vi "tempsave.vi"() -> ()   [LabVIEW 2014]
uses:
  <vilib>/rvi/DataTransferAndStorage/Container/XNode/niFpgaContainer.xnode
  <vilib>/rvi/FIFO/Fifo_Resource/niFpgaFifoEmulationRefIn.vi
  FPGA Function.ctl
panel:
  in  "PosVal 2":u32
  in  "SerialFunction 2":T1
  out "NOBWrite 2":i32
  in  "Delay W/R 2":u32=4
  out "Pos 2":u32
  out "Position":i32
  out "Pos 1":u32
  in  "PosVal":u32
  in  "SerialFunction":T1
  out "PresentPos":u64[](array[numeric])
  out "NOBWrite":i32
  in  "Delay W/R":u32=550
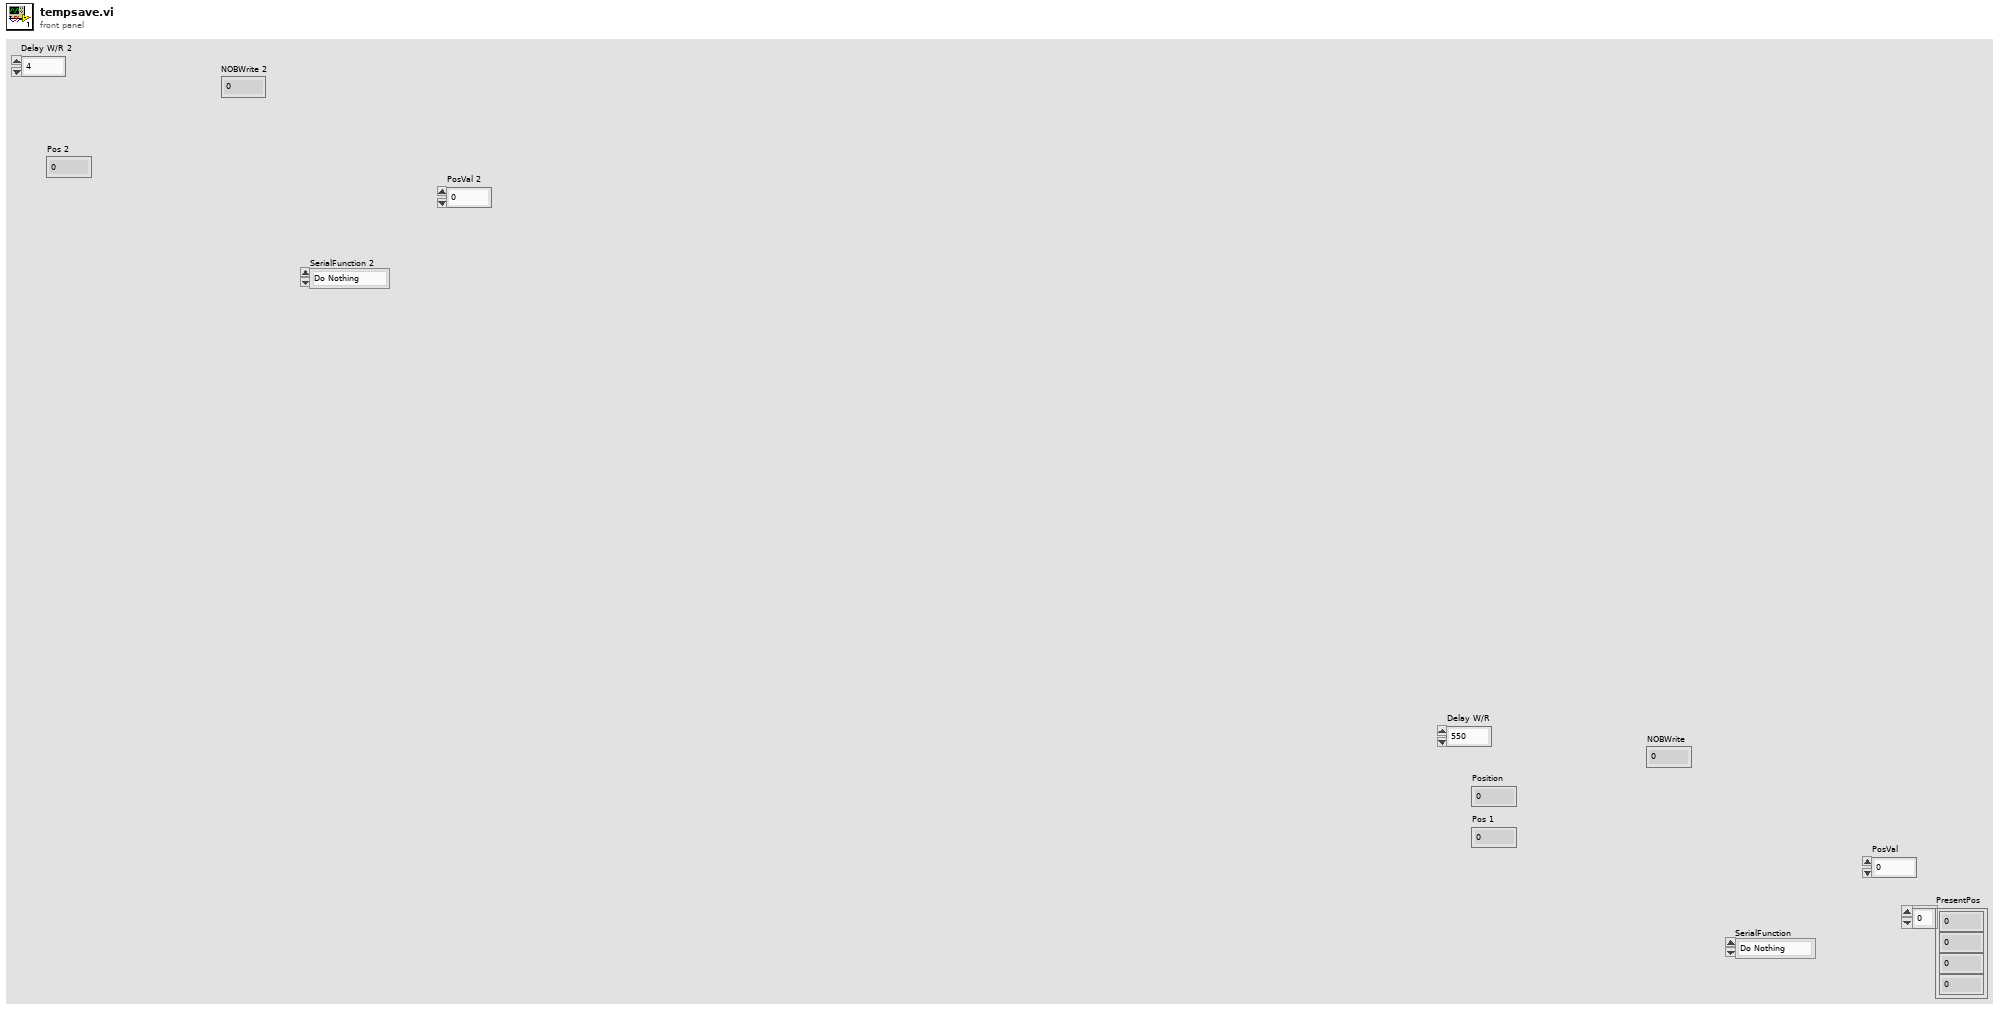
[diagram p1: front panel]
types:
  T1 = typedef "FPGA Function.ctl" = enum16{"Do Nothing", "Write", "Read"}
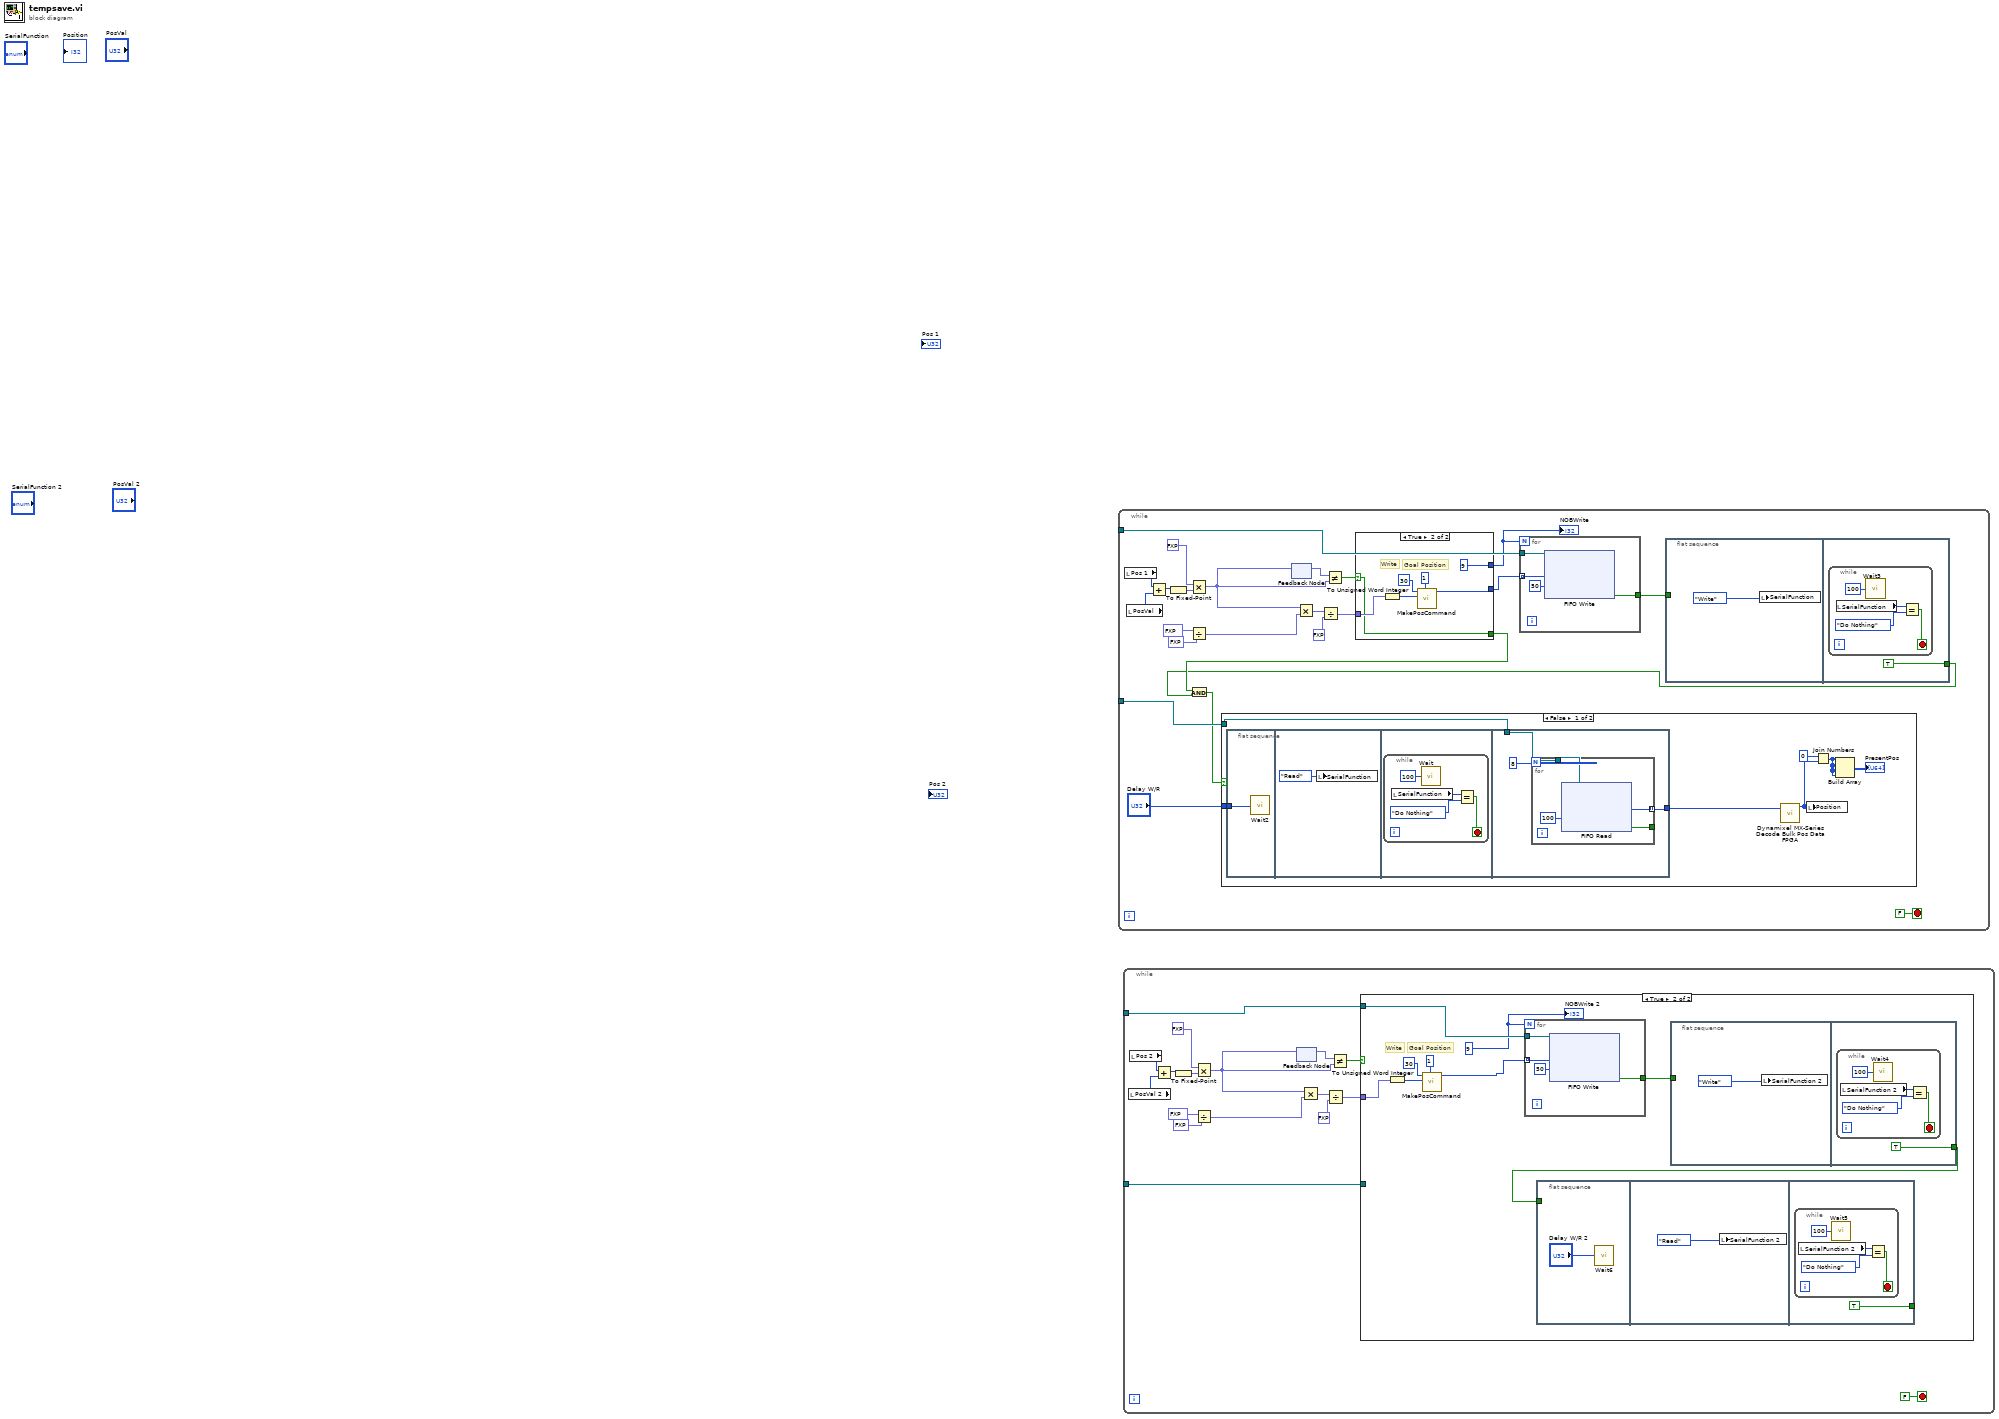
[diagram p0: block diagram]
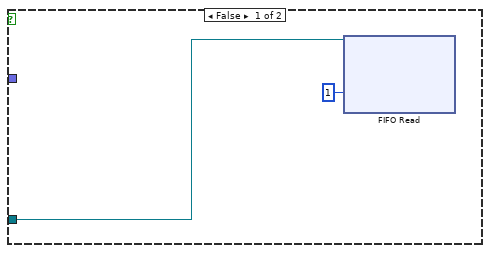
[diagram p2: hidden frame]
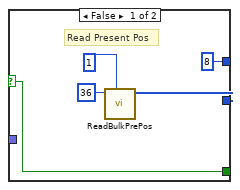
[diagram p4: hidden frame]
diagram:
  n1 = while {
    tunnel: _ -> [w9]
    tunnel: _ -> [w8]
    stop <- FALSE stop-if-true
    n2 = local read "Pos 1"() -> (w7:u32)
    n3 = local read "PosVal"() -> (w4:u32)
    n4 = Add(x=w7, y=w4) -> (x+y=w5:u32)
    n5 = To Fixed-Point(number=w5) -> (fixed-point=w19:fxp<+,32,32>)  [unwired: 1 in]
    n6 = Multiply(x=fxp<+,3,4> 10.0, y=w19) -> (x*y=w14:fxp<+,35,36>)
    n7 = Divide(x=fxp<+,12,12> 4095.0, y=fxp<+,6,9> 360.0) -> (x/y=w17:fxp<+,13,4>)
    n8 = feedback #1() -> (w15:fxp<+,35,36>)  [unwired: 1 in]
    n9 = feedback-in #1(w14) -> ()
    n10 = Multiply(x=w14, y=w17) -> (x*y=w21:fxp<+,47,39>)
    n11 = Divide(x=w21, y=fxp<+,3,4> 10.0) -> (x/y=w16:fxp<+,48,36>)
    n12 = Not Equal?(x=w15, y=w14) -> (x != y?=w13:bool)
    n13 = case shown="True" w13 {
      selector: w13 -> [w59 w62]
      tunnel: w16 -> [_ w63]
      tunnel: [w58 w61] -> w11
      tunnel: [w59 w62] -> w10
      tunnel: [8 9] -> w6
      frame False {
        # "Read Present Pos"
        n14 = call "ReadBulkPrePos.vi"(7:u8 1 ("MxID"), 11:u8 36 ("RegAddr")) -> ("Data"=w58:u8[])  [unwired: 8 in, 1 out]
      }
      frame True {
        # "Write"
        # "Goal Position"
        n15 = To Unsigned Word Integer(number=w63) -> (unsigned 16bit integer=w64:u16)
        n16 = call "MakePosCommand.vi"("MxID"=u8 1, "Param"=w64, "RegAddr"=u8 30) -> ("Data"=w61:u8[])  [unwired: 7 in, 1 out]
      }
    }
    "NOBWrite" <- w6
    n17 = And(x=w10, y=w2) -> (x .and. y?=w3:bool)
    n18 = case shown="False" w3 {
      tunnel: w8 -> [w37 _]
      tunnel: "Delay W/R" -> [w31 _]
      frame False {
        n19 = flat-sequence {
          tunnel: w31 -> [w38]
          tunnel: w37 -> [w46]
          tunnel: [w44] -> w36
          frame #0 {
            n20 = call "Wait2"("Count(uSec)"=w38) -> ()  [unwired: 1 out]
          }
          frame #1 {
            n21 = local write "SerialFunction"(FPGA_Function."Read" ("SerialFunction")) -> ()
          }
          frame #2 {
            n22 = while {
              stop <- w42 stop-if-true
              n23 = local read "SerialFunction"() -> (w41:T1)
              n24 = call "Wait"("Count(uSec)"=u32 100) -> ()  [unwired: 1 out]
              n25 = Equal?(x=w41, y=FPGA_Function."Do Nothing" ("SerialFunction")) -> (x = y?=w42:bool)
            }
          }
          frame #3 {
            n26 = for {
              N: 8 -> [_]
              tunnel: w46 -> [w50]
              tunnel: [w48] -> _
              tunnel: [w47] -> w44 mode=indexing
              n27 = xnode ("FIFO Read")("Timeout"=100, "FIFO In"=w50) -> ("Element"=w47:u8, "Timed Out?"=w48:bool)  [unwired: 1 out]
            }
          }
        }
        n28 = call "Dynamixel MX-Series Decode Bulk Pos Data FPGA.vi"("RecData"=w36) -> ("Position"=w35:u32[])  [unwired: 9 in, 1 out]
        n29 = local write "Position"(w35) -> ()
        n30 = Join Numbers(hi=0, lo=w35) -> ((hi.lo)=w32:u64[])
        n31 = Build Array(w32, w32, w32, w32) -> (→"PresentPos":u64[][])
      }
      frame True {
      }
    }
    n32 = for {
      N: w6 -> [_]
      tunnel: w9 -> [w54]
      tunnel: w11 -> [w53] mode=indexing
      tunnel: [w52] -> w12
      n33 = xnode ("FIFO Write")("FIFO In"=w54, "Element"=w53, "Timeout"=50) -> ("Timed Out?"=w52:bool)  [unwired: 1 out]
    }
    n34 = flat-sequence {
      tunnel: w12 -> [_]
      tunnel: [TRUE] -> w2
      frame #0 {
        n35 = local write "SerialFunction"(FPGA_Function."Write" ("Op Control")) -> ()
      }
      frame #1 {
        n36 = while {
          stop <- w29 stop-if-true
          n37 = local read "SerialFunction"() -> (w28:T1)
          n38 = call "Wait3"("Count(uSec)"=u32 100) -> ()  [unwired: 1 out]
          n39 = Equal?(x=w28, y=FPGA_Function."Do Nothing" ("SerialFunction")) -> (x = y?=w29:bool)
        }
      }
    }
  }
  n40 = while {
    tunnel: _ -> [w72]
    tunnel: _ -> [w67]
    stop <- FALSE stop-if-true
    n41 = local read "PosVal 2"() -> (w69:u32)
    n42 = local read "Pos 2"() -> (w71:u32)
    n43 = Add(x=w71, y=w69) -> (x+y=w70:u32)
    n44 = To Fixed-Point(number=w70) -> (fixed-point=w78:fxp<+,32,32>)  [unwired: 1 in]
    n45 = Multiply(x=fxp<+,3,4> 10.0, y=w78) -> (x*y=w73:fxp<+,35,36>)
    n46 = Divide(x=fxp<+,12,12> 4095.0, y=fxp<+,6,9> 360.0) -> (x/y=w76:fxp<+,13,4>)
    n47 = feedback #2() -> (w74:fxp<+,35,36>)  [unwired: 1 in]
    n48 = feedback-in #2(w73) -> ()
    n49 = Multiply(x=w73, y=w76) -> (x*y=w80:fxp<+,47,39>)
    n50 = Divide(x=w80, y=fxp<+,3,4> 10.0) -> (x/y=w75:fxp<+,48,36>)
    n51 = Not Equal?(x=w74, y=w73) -> (x != y?=w68:bool)
    n52 = case shown="True" w68 {
      tunnel: w75 -> [_ w94]
      tunnel: w72 -> [_ w91]
      tunnel: w67 -> [w85 _]
      frame False {
        n53 = xnode "FIFO Read"("Timeout"=1, "FIFO In"=w85) -> ()  [unwired: 3 out]
      }
      frame True {
        w90 = 9
        # "Write"
        # "Goal Position"
        n54 = To Unsigned Word Integer(number=w94) -> (unsigned 16bit integer=w87:u16)
        n55 = call "MakePosCommand.vi"("MxID"=u8 1, "Param"=w87, "RegAddr"=u8 30) -> ("Data"=w92:u8[])  [unwired: 7 in, 1 out]
        n56 = for {
          N: w90 -> [_]
          tunnel: w91 -> [w111]
          tunnel: w92 -> [w110] mode=indexing
          tunnel: [w109] -> w93
          n57 = xnode ("FIFO Write")("FIFO In"=w111, "Element"=w110, "Timeout"=50) -> ("Timed Out?"=w109:bool)  [unwired: 1 out]
        }
        n58 = flat-sequence {
          tunnel: w86 -> [_]
          tunnel: [TRUE] -> _
          frame #0 {
            n59 = call "Wait6"("Count(mSec)"="Delay W/R 2") -> ()  [unwired: 1 out]
          }
          frame #1 {
            n60 = local write "SerialFunction 2"(FPGA_Function."Read" ("Op Control")) -> ()
          }
          frame #2 {
            n61 = while {
              stop <- w100 stop-if-true
              n62 = local read "SerialFunction 2"() -> (w99:T1)
              n63 = call "Wait5"("Count(uSec)"=u32 100) -> ()  [unwired: 1 out]
              n64 = Equal?(x=w99, y=FPGA_Function."Do Nothing" ("SerialFunction")) -> (x = y?=w100:bool)
            }
          }
        }
        n65 = flat-sequence {
          tunnel: w93 -> [_]
          tunnel: [TRUE] -> w86
          frame #0 {
            n66 = local write "SerialFunction 2"(FPGA_Function."Write" ("Op Control")) -> ()
          }
          frame #1 {
            n67 = while {
              stop <- w106 stop-if-true
              n68 = local read "SerialFunction 2"() -> (w105:T1)
              n69 = call "Wait4"("Count(uSec)"=u32 100) -> ()  [unwired: 1 out]
              n70 = Equal?(x=w105, y=FPGA_Function."Do Nothing" ("SerialFunction")) -> (x = y?=w106:bool)
            }
          }
        }
        "NOBWrite 2" <- w90
      }
    }
  }
